vi "arrayconv.vi"(4 "Input 6":i32[](array[numeric]), 6 "Input 5":i32[](array[numeric]), 8 "Input 4":i32[](array[numeric]), 9 "Input 3":i32[](array[numeric]), 10 "Input 2":i32[](array[numeric]), 11 "Input 1":i32[](array[numeric])) -> (0 "output waveform 4":digitalwaveform(waveform)={"t0"=timestamp(0 s since 1904-01-01), "dt"=1.0, "Y"={"transitions"=[], "data"=[]}}, 1 "output waveform 3":digitalwaveform(waveform)={"t0"=timestamp(0 s since 1904-01-01), "dt"=1.0, "Y"={"transitions"=[], "data"=[]}}, 2 "output waveform 2":digitalwaveform(waveform)={"t0"=timestamp(0 s since 1904-01-01), "dt"=1.0, "Y"={"transitions"=[], "data"=[]}}, 3 "output waveform":digitalwaveform(waveform)={"t0"=timestamp(0 s since 1904-01-01), "dt"=1.0, "Y"={"transitions"=[], "data"=[]}}, 5 "output waveform 6":digitalwaveform(waveform)={"t0"=timestamp(0 s since 1904-01-01), "dt"=1.0, "Y"={"transitions"=[], "data"=[]}}, 7 "output waveform 5":digitalwaveform(waveform)={"t0"=timestamp(0 s since 1904-01-01), "dt"=1.0, "Y"={"transitions"=[], "data"=[]}})   [LabVIEW 2026]
uses:
  <vilib>/Waveform/DTblOps.llb/DTbl Boolean Array to Digital.vi
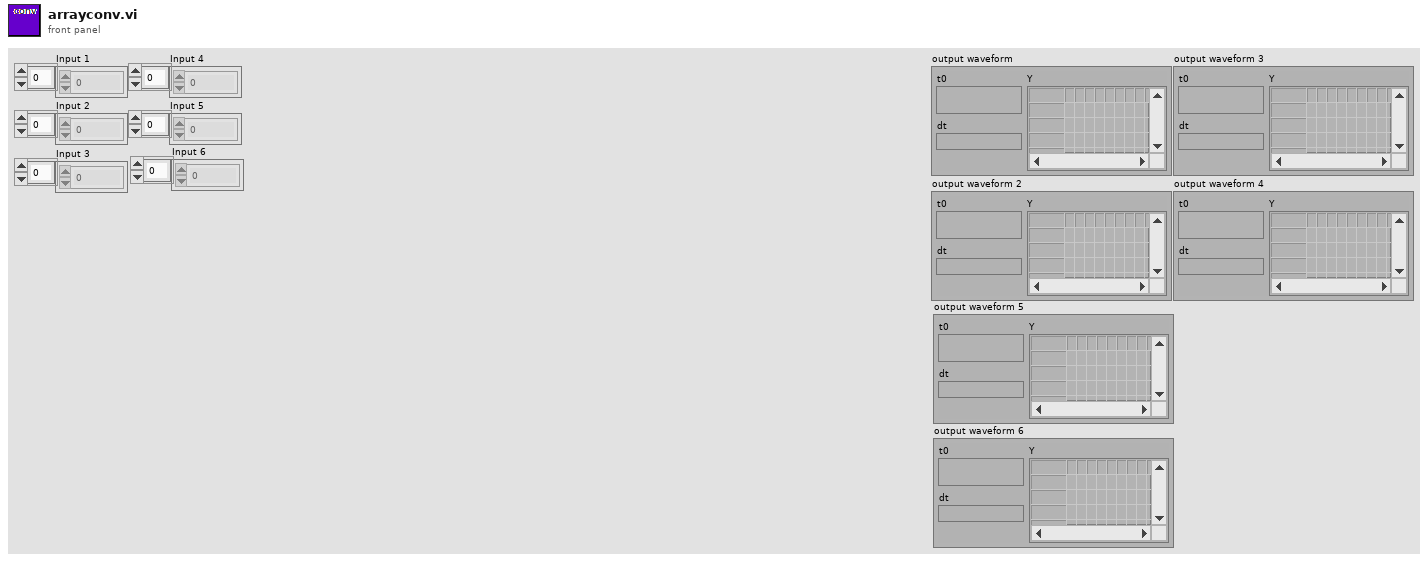
[diagram p1: front panel]
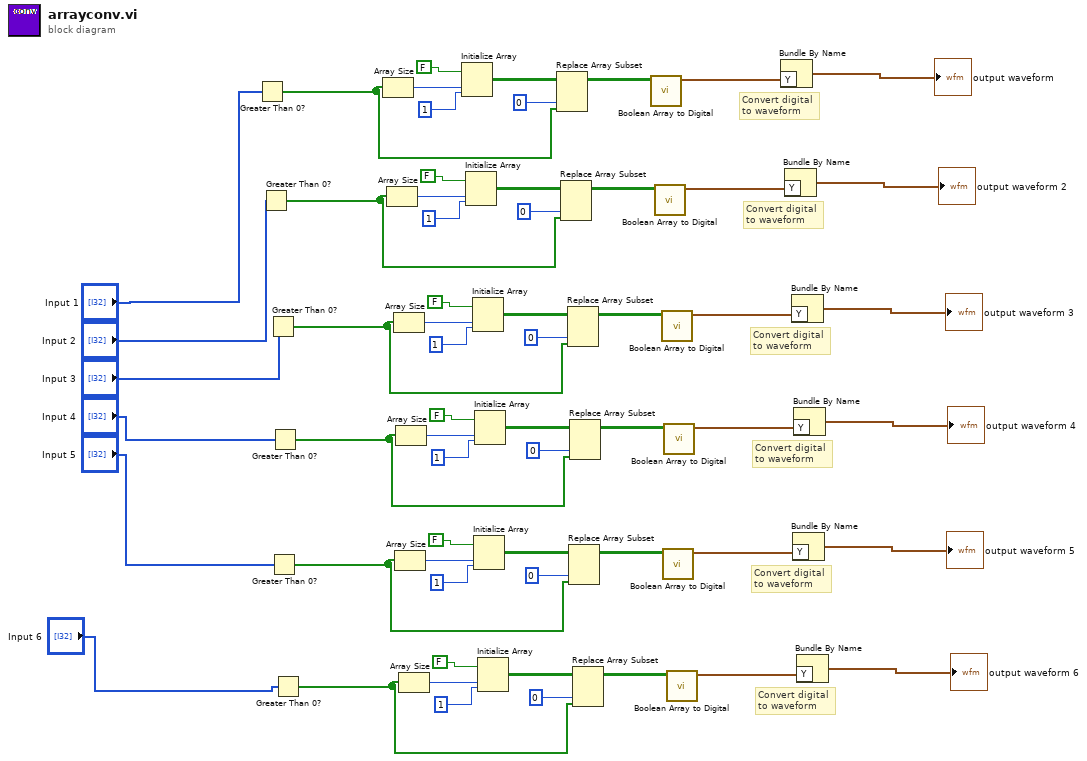
[diagram p0: block diagram]
diagram:
  # "Convert digital\nto waveform"
  # "Convert digital\nto waveform"
  # "Convert digital\nto waveform"
  # "Convert digital\nto waveform"
  # "Convert digital\nto waveform"
  # "Convert digital\nto waveform"
  n1 = Greater Than 0?(x="Input 1") -> (x > 0?=w53:bool[])
  n2 = Greater Than 0?(x="Input 2") -> (x > 0?=w49:bool[])
  n3 = Greater Than 0?(x="Input 3") -> (x > 0?=w34:bool[])
  n4 = Greater Than 0?(x="Input 5") -> (x > 0?=w16:bool[])
  n5 = Greater Than 0?(x="Input 4") -> (x > 0?=w31:bool[])
  n6 = Greater Than 0?(x="Input 6") -> (x > 0?=w13:bool[])
  n7 = Array Size(array=w53) -> (size(s)=w59:i32)
  n8 = Array Size(array=w49) -> (size(s)=w43:i32)
  n9 = Array Size(array=w34) -> (size(s)=w40:i32)
  n10 = Array Size(array=w16) -> (size(s)=w22:i32)
  n11 = Array Size(array=w31) -> (size(s)=w25:i32)
  n12 = Array Size(array=w13) -> (size(s)=w7:i32)
  n13 = Initialize Array(FALSE, w59, 1 ("dimension size")) -> (w60:bool[][])
  n14 = Initialize Array(FALSE, w43, 1 ("dimension size")) -> (w42:bool[][])
  n15 = Initialize Array(FALSE, w40, 1 ("dimension size")) -> (w41:bool[][])
  n16 = Initialize Array(FALSE, w22, 1 ("dimension size")) -> (w23:bool[][])
  n17 = Initialize Array(FALSE, w25, 1 ("dimension size")) -> (w24:bool[][])
  n18 = Initialize Array(FALSE, w7, 1 ("dimension size")) -> (w6:bool[][])
  n19 = Replace Array Subset(array=w60, new element=w53, index (col)=0 ("index (row)")) -> (w57:bool[][])  [unwired: 1 in]
  n20 = Replace Array Subset(array=w42, new element=w49, index (col)=0 ("index (row)")) -> (w45:bool[][])  [unwired: 1 in]
  n21 = Replace Array Subset(array=w41, new element=w34, index (col)=0 ("index (row)")) -> (w38:bool[][])  [unwired: 1 in]
  n22 = Replace Array Subset(array=w23, new element=w16, index (col)=0 ("index (row)")) -> (w20:bool[][])  [unwired: 1 in]
  n23 = Replace Array Subset(array=w24, new element=w31, index (col)=0 ("index (row)")) -> (w27:bool[][])  [unwired: 1 in]
  n24 = Replace Array Subset(array=w6, new element=w13, index (col)=0 ("index (row)")) -> (w9:bool[][])  [unwired: 1 in]
  n25 = call-poly <vilib>:"Boolean Array to Digital.vi"("boolean array"=w57) -> ("digital data"=w58:digitaldata)  [unwired: 3 in, 7 out]
  n26 = call-poly <vilib>:"Boolean Array to Digital.vi"("boolean array"=w45) -> ("digital data"=w44:digitaldata)  [unwired: 3 in, 7 out]
  n27 = call-poly <vilib>:"Boolean Array to Digital.vi"("boolean array"=w38) -> ("digital data"=w39:digitaldata)  [unwired: 3 in, 7 out]
  n28 = call-poly <vilib>:"Boolean Array to Digital.vi"("boolean array"=w20) -> ("digital data"=w21:digitaldata)  [unwired: 3 in, 7 out]
  n29 = call-poly <vilib>:"Boolean Array to Digital.vi"("boolean array"=w27) -> ("digital data"=w26:digitaldata)  [unwired: 3 in, 7 out]
  n30 = call-poly <vilib>:"Boolean Array to Digital.vi"("boolean array"=w9) -> ("digital data"=w8:digitaldata)  [unwired: 3 in, 7 out]
  n31 = Bundle By Name("Y"=w58) -> (→"output waveform":digitalwaveform)  [unwired: 1 in]
  n32 = Bundle By Name("Y"=w44) -> (→"output waveform 2":digitalwaveform)  [unwired: 1 in]
  n33 = Bundle By Name("Y"=w39) -> (→"output waveform 3":digitalwaveform)  [unwired: 1 in]
  n34 = Bundle By Name("Y"=w21) -> (→"output waveform 5":digitalwaveform)  [unwired: 1 in]
  n35 = Bundle By Name("Y"=w26) -> (→"output waveform 4":digitalwaveform)  [unwired: 1 in]
  n36 = Bundle By Name("Y"=w8) -> (→"output waveform 6":digitalwaveform)  [unwired: 1 in]
